vi "CameraCheckROI.vi"(8 "error in (no error)":errorcluster, 10 "ROI_in":T1, 11 "IMAQdx in":refnum<class "IMAQdx_Flea3_Firewire.lvclass">) -> (0 "error out":errorcluster, 2 "ROI_out":T1, 3 "IMAQdx out":refnum<class "IMAQdx_Flea3_Firewire.lvclass">)   [LabVIEW 2012, in "IMAQdx_Flea3_Firewire.lvclass"]
uses:
  <userlib>/BIAS2/classes/IMAQdx_Flea3_Firewire/IMAQdx_Flea3_Firewire.lvclass
  <userlib>/BIAS2/subvis/ROI_rect.ctl
  <userlib>/BIAS2/classes/IMAQdx_Flea3_Firewire/IMAQdx_Flea3_Firewire.lvclass/IMAQdx_Flea3_Firewire.ctl
  <resource>/objmgr/imaqdx.rc
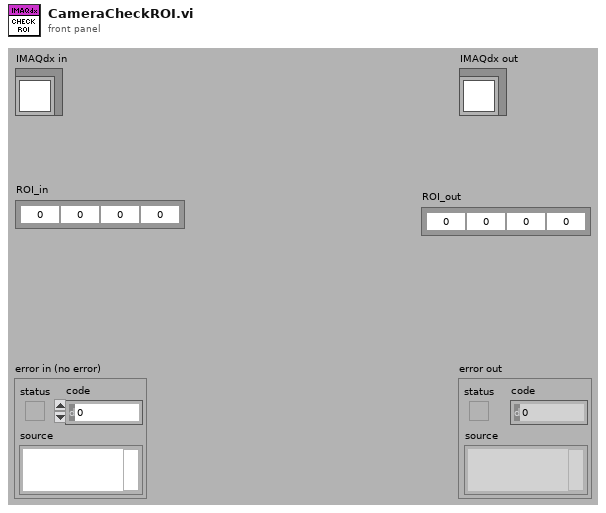
[diagram p1: front panel]
types:
  T1 = typedef "ROI_rect.ctl" = cluster{"left":i32, "top":i32, "right":i32, "bottom":i32}
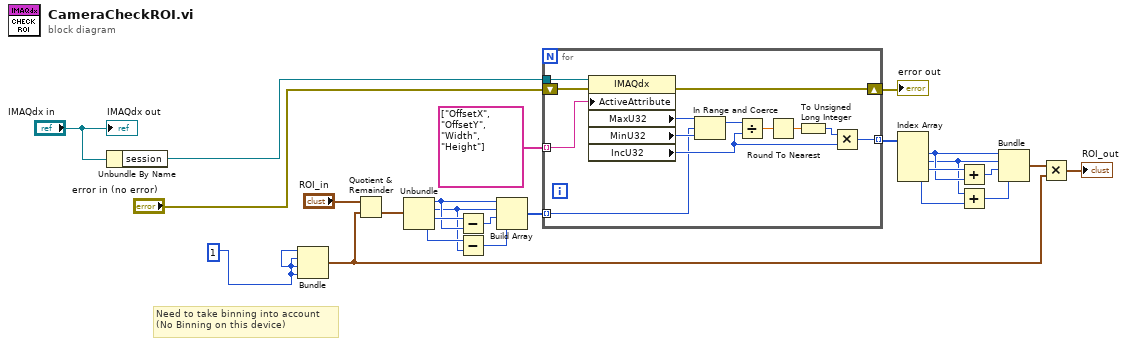
[diagram p0: block diagram]
diagram:
  w1 = 1
  # "Need to take binning into account\n(No Binning on this device)"
  n1 = Unbundle By Name("IMAQdx in") -> ("session"=w3:refnum<k21>)
  n2 = Bundle(w1, w1, w1, w1) -> (w4:cluster{i32, i32, i32, i32})  [unwired: 1 in]
  n3 = Quotient & Remainder(x="ROI_in", y=w4) -> (floor(x/y)=w7:T1)  [unwired: 1 out]
  n4 = Unbundle(w7) -> ("left"=w23:i32, "top"=w22:i32, "right"=w25:i32, "bottom"=w24:i32)
  n5 = Subtract(x=w25, y=w23) -> (x-y=w21:i32)
  n6 = Subtract(x=w24, y=w22) -> (x-y=w20:i32)
  n7 = Build Array(w23, w22, w21, w20) -> (w19:i32[])
  n8 = for {
    tunnel: w19 -> [w26] mode=indexing
    tunnel: string[] ["OffsetX", "OffsetY", "Width", "Height"] -> [w36] mode=indexing
    shift-right: [w38] -> w16
    shift-left: "error in (no error)" -> [w37]
    tunnel: w3 -> [w35]
    tunnel: [w27] -> w15 mode=indexing
    n9 = property class="IMAQdx"(reference=w35, error in=w37, "ActiveAttribute"=w36) -> (error out=w38:errorcluster, "MaxU32"=w32:u32, "MinU32"=w31:u32, "IncU32"=w28:u32)  [unwired: 1 out]
    n10 = In Range and Coerce(upper limit=w32, x=w26, lower limit=w31) -> (coerced(x)=w34:u32)  [unwired: 1 out]
    n11 = Divide(x=w34, y=w28) -> (x/y=w33:dbl)
    n12 = Round To Nearest(number=w33) -> (nearest integer value=w30:dbl)
    n13 = To Unsigned Long Integer(number=w30) -> (unsigned 32bit integer=w29:u32)
    n14 = Multiply(x=w29, y=w28) -> (x*y=w27:u32)
  }
  "error out" <- w16
  n15 = Index Array(array=w15) -> (element #1=w12:u32, element #2=w11:u32, element #3=w14:u32, element #4=w13:u32)  [unwired: 4 in]
  n16 = Add(x=w14, y=w12) -> (x+y=w10:u32)
  n17 = Add(x=w11, y=w13) -> (x+y=w9:u32)
  n18 = Bundle(w12, w11, w10, w9) -> (w6:cluster{u32, u32, u32, u32})  [unwired: 1 in]
  n19 = Multiply(x=w6, y=w4) -> (x*y=→"ROI_out":cluster{u32, u32, u32, u32})
  "IMAQdx out" <- "IMAQdx in"
